vi "IsHotGoal.vi"(8 "error in":errorcluster, 9 "% Cutoff":dbl, 10 "Num samples":i32) -> (0 "error out":errorcluster, 2 "Hot/Not":bool)   [LabVIEW 2013]
uses:
  Robot Global Data.vi
panel:
  out "x-y":u32
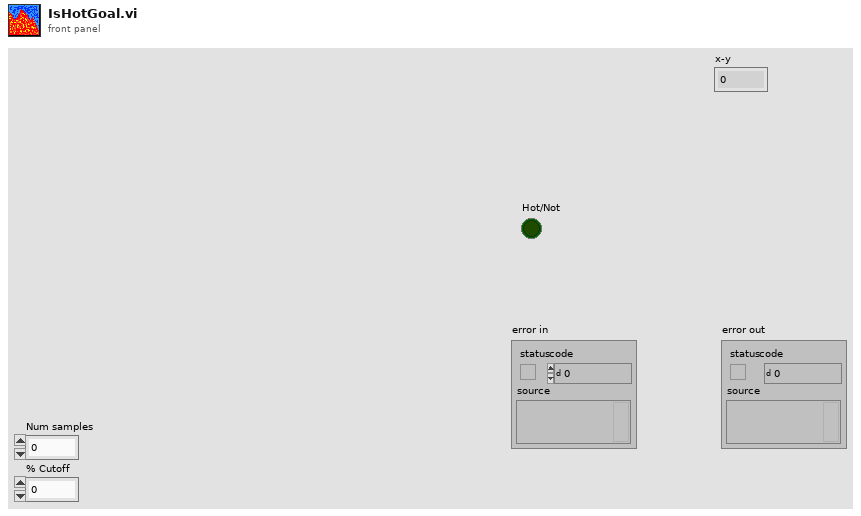
[diagram p1: front panel]
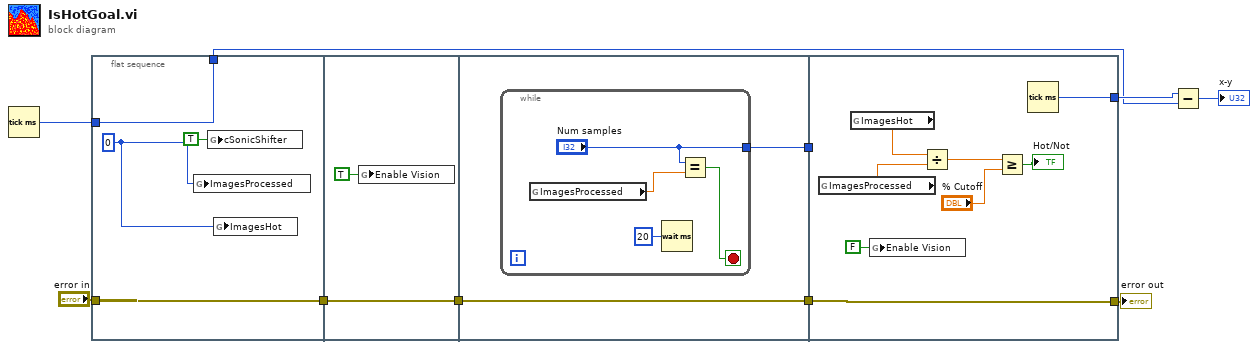
[diagram p0: block diagram]
diagram:
  n1 = Tick Count (ms)() -> (millisecond timer value=w4:u32)
  n2 = flat-sequence {
    tunnel: [w14] -> w6
    tunnel: "error in" -> [w14]
    tunnel: w4 -> [w12]
    tunnel: [w12] -> w2
    tunnel: w6 -> [w16]
    tunnel: [w16] -> w5
    tunnel: [w18] -> w10
    tunnel: w5 -> [w17]
    tunnel: [w17] -> w8
    tunnel: w10 -> [_]
    tunnel: w8 -> [w25]
    tunnel: [w25] -> w7
    tunnel: [w24] -> w3
    frame #0 {
      w13 = 0 ("Numeric")
      n3 = global write "Robot Global Data.vi" "ImagesProcessed"(w13) -> ()
      n4 = global write "Robot Global Data.vi" "cSonicShifter"(TRUE ("Enable Vision")) -> ()
      n5 = global write "Robot Global Data.vi" "ImagesHot"(w13) -> ()
    }
    frame #1 {
      n6 = global write "Robot Global Data.vi" "Enable Vision"(TRUE ("Enable Vision")) -> ()
    }
    frame #2 {
      n7 = while {
        tunnel: ["Num samples"] -> w18
        stop <- w21 stop-if-true
        n8 = global read "Robot Global Data.vi" "ImagesProcessed"() -> (w22:dbl)
        n9 = Wait (ms)(milliseconds to wait=u32 20) -> ()  [unwired: 1 out]
        n10 = Equal?(x="Num samples", y=w22) -> (x = y?=w21:bool)
      }
    }
    frame #3 {
      n11 = global read "Robot Global Data.vi" "ImagesProcessed"() -> (w23:dbl)
      n12 = global read "Robot Global Data.vi" "ImagesHot"() -> (w27:dbl)
      n13 = global write "Robot Global Data.vi" "Enable Vision"(FALSE ("Enable Vision")) -> ()
      n14 = Divide(x=w27, y=w23) -> (x/y=w30:dbl)
      n15 = Greater Or Equal?(x=w30, y="% Cutoff") -> (x >= y?=→"Hot/Not":bool)
      n16 = Tick Count (ms)() -> (millisecond timer value=w24:u32)
    }
  }
  n17 = Subtract(x=w3, y=w2) -> (x-y=→"x-y":u32)
  "error out" <- w7
